vi "Encoder State.vi"(8 "error in (no error)":errorcluster) -> (0 "error out":errorcluster, 2 "Gamma":dbl, 3 "Combined Wheel Angle":dbl)   [LabVIEW 2014]
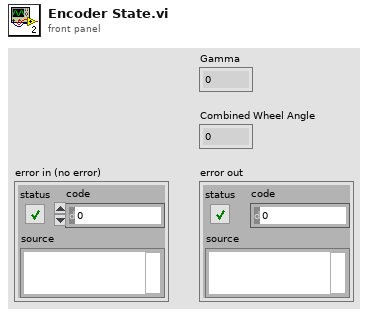
[diagram p1: front panel]
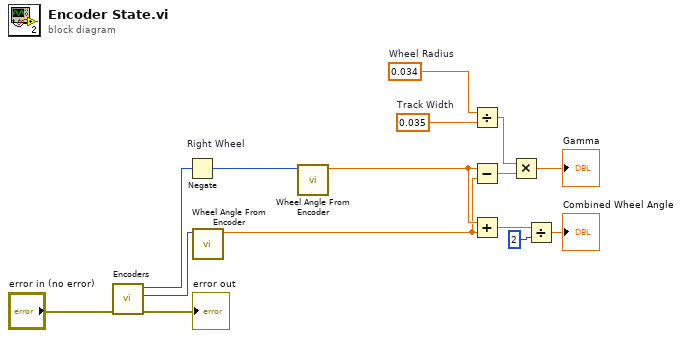
[diagram p0: block diagram]
diagram:
  w14 = 0.035  # Track Width
  w13 = 0.034  # Wheel Radius
  n1 = call "Encoders.vi"("error in (no error)"="error in (no error)") -> ("error out"=→"error out":errorcluster, "Encoder 3"=w9:i32, "Encoder 2"=w8:i32)  [unwired: 6 in, 2 out]
  n2 = Negate "Right Wheel"(x=w8) -> (-x=w7:i32)
  n3 = call "Wheel Angle From Encoder.vi"("Numeric in"=w9) -> ("Numeric out"=w10:dbl)  [unwired: 10 in]
  n4 = call "Wheel Angle From Encoder.vi"("Numeric in"=w7) -> ("Numeric out"=w11:dbl)  [unwired: 10 in]
  n5 = Divide(x=w13, y=w14) -> (x/y=w15:dbl)
  n6 = Subtract(x=w11, y=w10) -> (x-y=w2:dbl)
  n7 = Add(x=w11, y=w10) -> (x+y=w4:dbl)
  n8 = Multiply(x=w15, y=w2) -> (x*y=→"Gamma":dbl)
  n9 = Divide(x=w4, y=2) -> (x/y=→"Combined Wheel Angle":dbl)
